vi "ToString.vi"(8 "error in (no error)":errorcluster, 11 "IsEqual in":refnum<class "IsEqual.lvclass">) -> (0 "error out":errorcluster, 2 "String":string, 3 "IsEqual out":refnum<class "IsEqual.lvclass">)   [LabVIEW 2019, in "Constraint.lvlib" / "IsEqual.lvclass"]
doc: "Returns a string representation of the object."
uses:
  IsEqual.lvclass
  IsEqual.lvclass/IsEqual.ctl
  63865889-f0df-4046-9aee-ce1fe68c83e2.vi
  <vilib>/JDP Science/JSONtext/Variant to JSON Text.vi
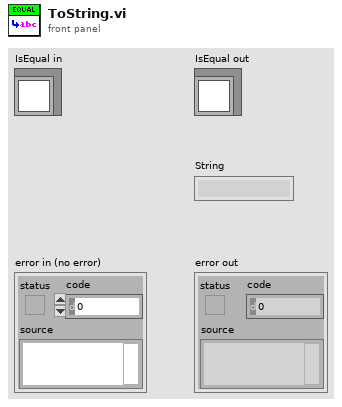
[diagram p1: front panel]
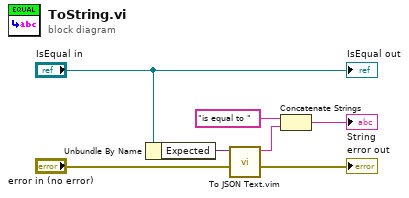
[diagram p0: block diagram]
diagram:
  n1 = Unbundle By Name("IsEqual in") -> ("Expected"=w3:variant)
  n2 = call "To JSON Text.vim"("error in (no error)"="error in (no error)", "Anything"=w3) -> ("error out"=→"error out":errorcluster, "<JSON>"=w1:string)  [unwired: 8 in]
  n3 = Concatenate Strings("is equal to " ("String"), w1) -> (→"String":string)
  "IsEqual out" <- "IsEqual in"
